vi "Main.vi"(11 "Module Admin":refnum<class "Delacor_lib_QMH_Cloneable Module Admin.lvclass">) -> ()   [LabVIEW 2020, in "Osciloscope.lvlib"]
doc: "This template is based off of the Queued Message Handler design pattern and the Queued Message Handler project template that ships with LabVIEW.\n\nThe main difference is that the queue is private to this module and communication between modules is performed via Broadcast and Request events.\n\nRequest events are wrapped in public API methods and are handled in the Event Handling Loop (EHL) of this VI. Any module can register for Broadcast events sent by this module. The EHL generates messages based on user interface actions.\n\nThe Message Handling Loop (MHL) processes messages generated by the EHL, or by other messages. The messages are string values, so new messages can be added easily to the Message Cases case structure in the MHL. Each message cluster can also provide an optional value for Message Data, which is a variant that can be converted to whatever message-specific data is required.\n_____\nBased on DQMH Project Template 6.0.0.91."
uses:
  Osciloscope.lvlib
  <vilib>/Delacor/Delacor QMH/Libraries/Cloneable Module Admin_class/Delacor_lib_QMH_Cloneable Module Admin.lvclass
  C:/Program Files (x86)/National Instruments/LabVIEW 2020/vi.lib/Delacor/Delacor QMH/Libraries/Module Admin_class/Delacor_lib_QMH_Module Admin.lvclass
  Module Data--cluster.ctl
  Classes/Osciloscope/Osciloscope.lvclass
  <vilib>/Delacor/Delacor QMH/Libraries/Message Queue_class/Delacor_lib_QMH_Message Queue.lvclass/Delacor_lib_QMH_Message Queue.ctl
  <vilib>/Delacor/Delacor QMH/Libraries/Cloneable Module Admin_class/Delacor_lib_QMH_Cloneable Module Admin.lvclass/Delacor_lib_QMH_Cloneable Module Admin.ctl
  Stop Argument--cluster.ctl
  <vilib>/Delacor/Delacor QMH/Libraries/Module Admin_class/Delacor_lib_QMH_Module Admin.lvclass/Delacor_lib_QMH_Module Admin.ctl
  Set Port Com Argument--cluster.ctl
  InicializarOsciloscopio Argument--cluster.ctl
  InitMethod Argument--cluster.ctl
  CloseMethod Argument--cluster.ctl
  MethodAutosetup Argument--cluster.ctl
  Method Configure Channel Argument--cluster.ctl
  Read Measurement Method Argument--cluster.ctl
  <vilib>/Utility/miscctls.llb/LVPointTypeDef.ctl
  Classes/Osciloscope/Osciloscope.lvclass/Osciloscope.ctl
  <vilib>/Delacor/Delacor QMH/Libraries/Message Queue_class/Delacor_lib_QMH_Enqueue Message (Single).vi
  <vilib>/Delacor/Delacor QMH/Libraries/Cloneable Module Admin_class/Delacor_lib_QMH_Get Module ID.vi
  <vilib>/Delacor/Delacor QMH/Libraries/Module Admin_class/Delacor_lib_QMH_Get External Launch.vi
  Classes/Osciloscope/Write COM.vi
  <vilib>/Utility/error.llb/Error Cluster From Error Code.vi
  <vilib>/ErrorRing/Error Ring.xnode
  <vilib>/Delacor/Delacor QMH/Libraries/Message Queue_class/Delacor_lib_QMH_Message Queue.lvclass
panel:
  out "error out":errorcluster
  out "Status":string
  in  "Simulate EHL Error":bool
  in  "Simulate MHL Error":bool
  # "Other QMH Modules communicate with this Module via its Public API (wrappers for its Request Events).\n\nThis Module communicates with other Modules via its Broadcast Events.\nAny module that wants to get these messages, just registers for this module's Broadcast events."
  # "This template is for the Delacor Modified Queued Message Handler design pattern.\n\nSee the block diagram for more information on how to use this template."
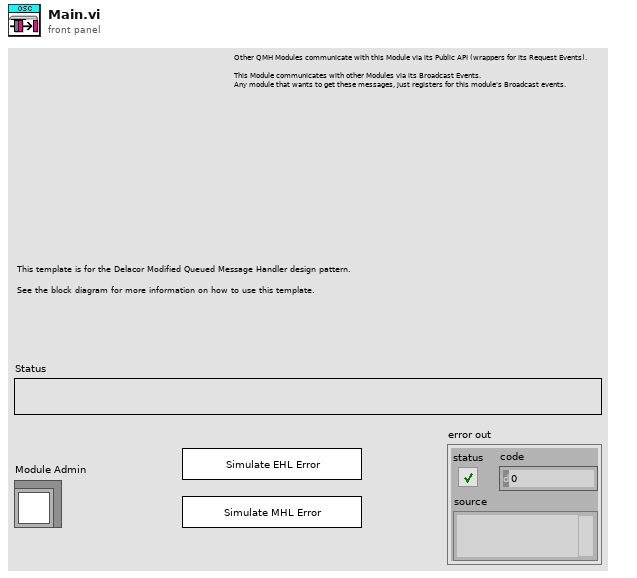
[diagram p1: front panel]
types:
  T1 = typedef "Osciloscope.lvlib/Request Events--cluster.ctl" = cluster{"Stop Module":refnum<user-event>, "Show Panel":refnum<user-event>, "Hide Panel":refnum<user-event>, "Show Diagram":refnum<user-event>, "Get Module Execution Status":refnum<user-event>, "Set Port Com":refnum<user-event>, "InicializarOsciloscopio":refnum<user-event>, "InitMethod":refnum<user-event>, "CloseMethod":refnum<user-event>, "MethodAutosetup":refnum<user-event>, "Method Configure Channel":refnum<user-event>, "Read Measurement Method":refnum<user-event>}
  T2 = typedef "Osciloscope.lvlib/Module Data--cluster.ctl" = cluster{"Status":string, "Com":refnum<visa-resource-name>, "Osciloscope.lvclass":refnum<class "Osciloscope.lvclass">}
  T3 = enum32{"invalid lock state", "Not Locked", "Locked (No Password)", "Password-protected"}
  T4 = typedef "Osciloscope.lvlib/Stop Argument--cluster.ctl" = cluster{"Module ID":i32, "Origin":string, "Exit via Stop Module Req?":bool, "Wait for Module to stop?":bool}
  T5 = typedef "Osciloscope.lvlib/Set Port Com Argument--cluster.ctl" = cluster{"Module ID":i32, "COM":refnum<visa-resource-name>}
  T6 = typedef "Osciloscope.lvlib/InicializarOsciloscopio Argument--cluster.ctl" = cluster{"Module ID":i32, "OsciloscopioName":string}
  T7 = typedef "Osciloscope.lvlib/InitMethod Argument--cluster.ctl" = cluster{"Module ID":i32, "Boolean":bool}
  T8 = typedef "Osciloscope.lvlib/CloseMethod Argument--cluster.ctl" = cluster{"Module ID":i32, "Boolean":bool}
  T9 = typedef "Osciloscope.lvlib/MethodAutosetup Argument--cluster.ctl" = cluster{"Module ID":i32, "Boolean":bool}
  T10 = typedef "Osciloscope.lvlib/Method Configure Channel Argument--cluster.ctl" = cluster{"Module ID":i32, "Boolean":bool}
  T11 = typedef "Osciloscope.lvlib/Read Measurement Method Argument--cluster.ctl" = cluster{"Module ID":i32, "Boolean":bool}
  T12 = typedef "LVPointTypeDef.ctl" = cluster{"Horizontal":i16, "Vertical":i16}
  T13 = enum32{"Invalid", "Standard", "Closed", "Hidden", "Minimized", "Maximized"}
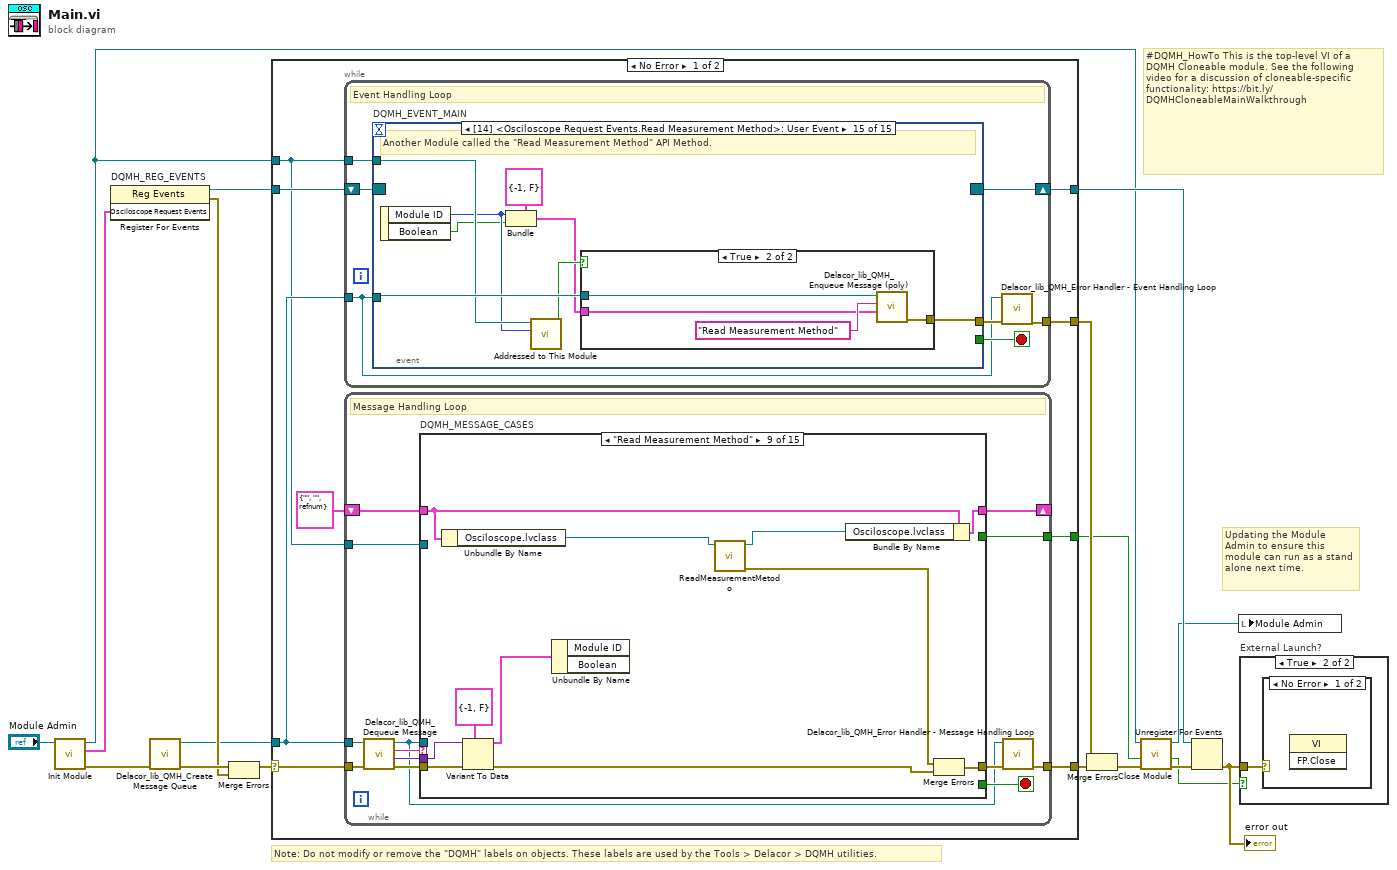
[diagram p0: block diagram]
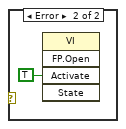
[diagram p3: hidden frame]
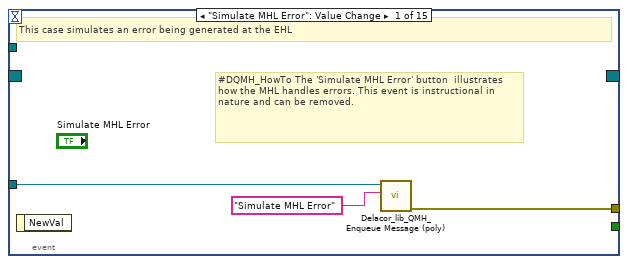
[diagram p4: hidden frame]
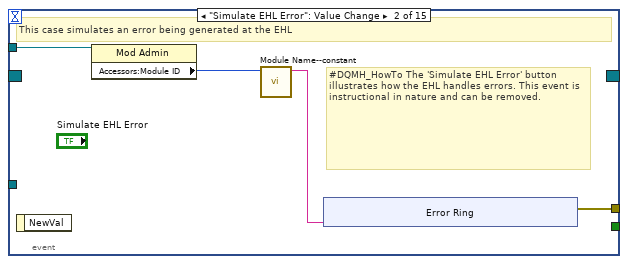
[diagram p5: hidden frame]
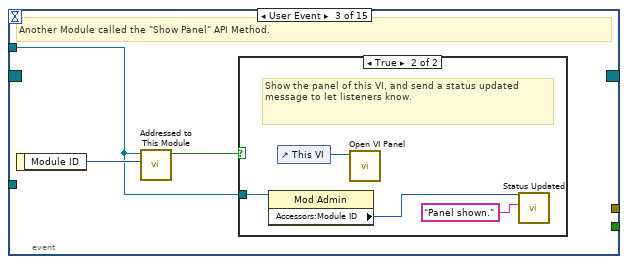
[diagram p6: hidden frame]
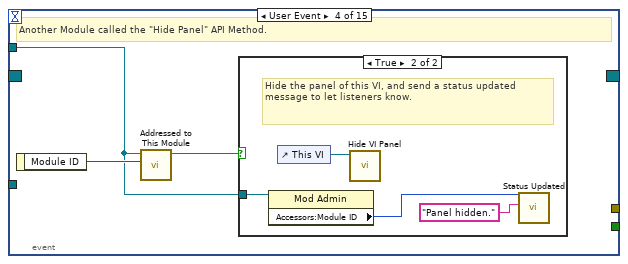
[diagram p8: hidden frame]
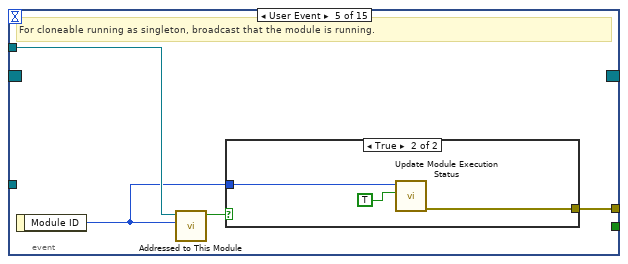
[diagram p10: hidden frame]
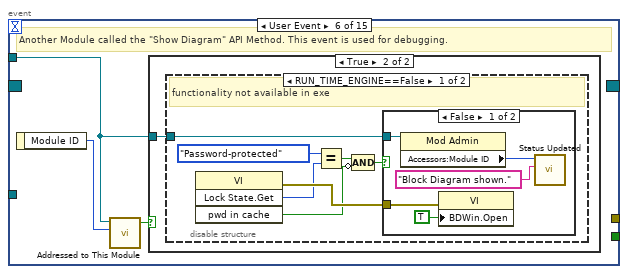
[diagram p12: hidden frame]
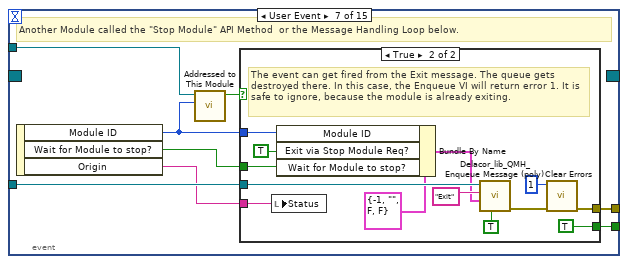
[diagram p16: hidden frame]
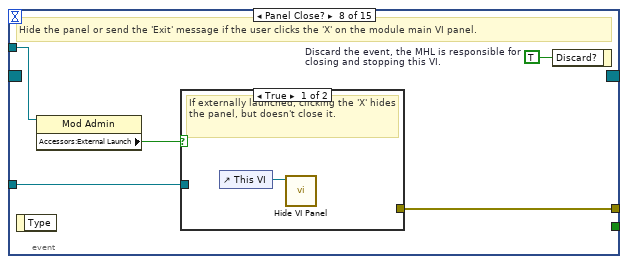
[diagram p18: hidden frame]
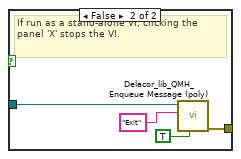
[diagram p19: hidden frame]
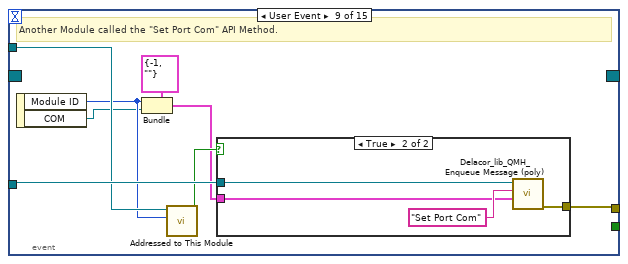
[diagram p20: hidden frame]
diagram:
  # "#DQMH_HowTo This is the top-level VI of a DQMH Cloneable module. See the following video for a discussion of cloneable-specific functionality: https://bit.ly/DQMHCloneableMainWalkthrough"
  # "Note: Do not modify or remove the \"DQMH\" labels on objects. These labels are used by the Tools > Delacor > DQMH utilities."
  # "Updating the Module Admin to ensure this module can run as a stand alone next time."
  n1 = call "Init Module.vi"("Cloneable Module Admin in"="Module Admin") -> ("error out"=w15:errorcluster, "Osciloscope Request Events"=w7:T1, "Cloneable Module Admin out"=w4:refnum<class "Delacor_lib_QMH_Cloneable Module Admin.lvclass">)  [unwired: 8 in]
  n2 = register-events "DQMH_REG_EVENTS"(w7) -> (reference out=w8:refnum<event-registration>, error out=w10:errorcluster)  [unwired: 2 in]
  n3 = call <vilib>:"Delacor_lib_QMH_Create Message Queue.vi"("error in"=w15) -> ("error out"=w12:errorcluster, "Message Queue"=w6:refnum<class "Delacor_lib_QMH_Message Queue.lvclass">)  [unwired: 9 in]
  n4 = Merge Errors(w12, w10) -> (w11:errorcluster)
  n5 = case shown="No Error" w11 {
    selector: w11 -> [w25 w384]
    tunnel: [w27 w383] -> w16
    tunnel: [w24 w391] -> w9
    tunnel: w8 -> [w22 w391]
    tunnel: w6 -> [w21 w382]
    tunnel: [w26 _] -> w17
    tunnel: w4 -> [w20 w387]
    tunnel: [w19 _] -> w2
    frame No Error {
      n6 = while {
        tunnel: w21 -> [w28]
        shift-right: [w31] -> w24
        shift-left: w22 -> [w32]
        tunnel: [w33] -> w26
        tunnel: w20 -> [w29]
        stop <- w30 stop-if-true
        # "Event Handling Loop"
        n7 = event "DQMH_EVENT_MAIN" shown="[14] <Osciloscope Request Events.Read Measurement Method>: User Event" {
          selector: w32 -> [_ _ _ _ _ _ _ _ _ _ _ _ _ _ _]
          dyn-events: [_ _ _ _ _ _ _ _ _ _ _ _ _ _ _] -> w31
          timeout: _ -> [_ _ _ _ _ _ _ _ _ _ _ _ _ _ _]
          tunnel: [_ _ _ _ _ _ w89 _ _ _ _ _ _ _ _] -> w30
          tunnel: w28 -> [w36 _ _ _ _ _ w92 w108 w124 w136 w148 w160 w172 w184 w196]
          tunnel: [w37 w41 _ _ w66 _ w93 w111 w117 w129 w141 w153 w165 w177 w189] -> w34
          tunnel: w29 -> [_ w40 w49 w56 w64 w70 w91 w109 w122 w134 w146 w158 w170 w182 w194]
          event "Simulate MHL Error": Value Change {
            # "#DQMH_HowTo The 'Simulate MHL Error' button  illustrates how the MHL handles errors. This event is instructional in nature and can be removed."
            # "This case simulates an error being generated at the EHL"
            n8 = event-data() -> ()  [unwired: 1 in, 1 out]
            n9 = call-poly <vilib>:"Delacor_lib_QMH_Enqueue Message (poly).vi"("Message"="Simulate MHL Error", "Message Queue in"=w36) -> ("error out"=w37:errorcluster)  [unwired: 8 in, 1 out]
          }
          event "Simulate EHL Error": Value Change {
            # "#DQMH_HowTo The 'Simulate EHL Error' button  illustrates how the EHL handles errors. This event is instructional in nature and can be removed."
            # "This case simulates an error being generated at the EHL"
            n10 = event-data() -> ()  [unwired: 1 in, 1 out]
            n11 = property class="Mod Admin"(reference=w40) -> ("Accessors:Module ID"=w39:i32)  [unwired: 1 in, 2 out]
            n12 = call "Module Name--constant.vi"("Module ID"=w39) -> ("Module Name"=w38:string)  [unwired: 10 in]
            n13 = xnode "Error Ring"("parameter 0"=w38) -> ("error out"=w41:errorcluster)
          }
          event User Event {
            # "Another Module called the \"Show Panel\" API Method."
            n14 = event-data() -> ("Module ID"=w50:i32)  [unwired: 1 in]
            n15 = call "Addressed to This Module.vi"("Module ID from Argument"=w50, "Module Admin"=w49) -> ("Addressed to this instance?"=w51:bool)  [unwired: 8 in, 1 out]
            n16 = case shown="True" w51 {
              tunnel: w49 -> [_ w53]
              frame False {
              }
              frame True {
                # "Show the panel of this VI, and send a status updated message to let listeners know."
                n17 = property class="Mod Admin"(reference=w53) -> ("Accessors:Module ID"=w52:i32)  [unwired: 1 in, 2 out]
                n18 = control-ref of="This VI"() -> (w55:refnum<vi>)
                n19 = call "Open VI Panel.vi"("VI"=w55) -> ()  [unwired: 10 in, 1 out]
                n20 = call "Status Updated.vi"("Status"="Panel shown." ("format string"), "Module ID"=w52) -> ()  [unwired: 9 in, 1 out]
              }
            }
          }
          event User Event {
            # "Another Module called the \"Hide Panel\" API Method."
            n21 = event-data() -> ("Module ID"=w57:i32)  [unwired: 1 in]
            n22 = call "Addressed to This Module.vi"("Module ID from Argument"=w57, "Module Admin"=w56) -> ("Addressed to this instance?"=w58:bool)  [unwired: 8 in, 1 out]
            n23 = case shown="True" w58 {
              tunnel: w56 -> [_ w60]
              frame False {
              }
              frame True {
                # "Hide the panel of this VI, and send a status updated message to let listeners know."
                n24 = property class="Mod Admin"(reference=w60) -> ("Accessors:Module ID"=w59:i32)  [unwired: 1 in, 2 out]
                n25 = control-ref of="This VI"() -> (w62:refnum<vi>)
                n26 = call "Hide VI Panel.vi"("VI"=w62) -> ()  [unwired: 10 in, 1 out]
                n27 = call "Status Updated.vi"("Status"="Panel hidden." ("format string"), "Module ID"=w59) -> ()  [unwired: 9 in, 1 out]
              }
            }
          }
          event User Event {
            # "For cloneable running as singleton, broadcast that the module is running."
            n28 = event-data() -> ("Module ID"=w63:i32)  [unwired: 1 in]
            n29 = call "Addressed to This Module.vi"("Module ID from Argument"=w63, "Module Admin"=w64) -> ("Addressed to this instance?"=w65:bool)  [unwired: 8 in, 1 out]
            n30 = case shown="True" w65 {
              tunnel: [_ w69] -> w66
              tunnel: w63 -> [_ w68]
              frame False {
              }
              frame True {
                n31 = call "Update Module Execution Status.vi"("Running?"=TRUE, "Module ID"=w68) -> ("error out"=w69:errorcluster)  [unwired: 9 in]
              }
            }
          }
          event User Event {
            # "Another Module called the \"Show Diagram\" API Method. This event is used for debugging."
            n32 = event-data() -> ("Module ID"=w71:i32)  [unwired: 1 in]
            n33 = call "Addressed to This Module.vi"("Module ID from Argument"=w71, "Module Admin"=w70) -> ("Addressed to this instance?"=w72:bool)  [unwired: 8 in, 1 out]
            n34 = case shown="True" w72 {
              tunnel: w70 -> [_ w73]
              frame False {
              }
              frame True {
                n35 = disable-structure shown="RUN_TIME_ENGINE==False" {
                  disable-tunnel: w73 -> [w74 _]
                  frame condition #0 (active) {
                    # "functionality not available in exe"
                    n36 = invoke class="VI" method="Lock State.Get"() -> (error out=w80:errorcluster, "Get Lock State"=w79:T3, "pwd in cache"=w76:bool)  [unwired: 4 in, 1 out]
                    n37 = Equal?(x=T3."Password-protected", y=w79) -> (x = y?=w77:bool)
                    n38 = Compound Arithmetic op=AND(w77, invert w76) -> (w75:bool)
                    n39 = case shown="False" w75 {
                      tunnel: w80 -> [w85 _]
                      tunnel: w74 -> [w82 _]
                      frame False {
                        n40 = property class="Mod Admin"(reference=w82) -> ("Accessors:Module ID"=w81:i32)  [unwired: 1 in, 2 out]
                        n41 = property class="VI"(error in=w85, "BDWin.Open"=TRUE ("Block Diagram Window:Open")) -> ()  [unwired: 1 in, 2 out]
                        n42 = call "Status Updated.vi"("Status"="Block Diagram shown." ("format string"), "Module ID"=w81) -> ()  [unwired: 9 in, 1 out]
                      }
                      frame True {
                        # "Password-protected VI, and the password is not in the cache. Do not show the diagram."
                      }
                    }
                  }
                  frame condition #1 {
                  }
                }
              }
            }
          }
          event User Event {
            # "Another Module called the \"Stop Module\" API Method  or the Message Handling Loop below."
            n43 = event-data() -> ("Module ID"=w87:i32, "Wait for Module to stop?"=w88:bool, "Origin"=w86:string)  [unwired: 1 in]
            n44 = call "Addressed to This Module.vi"("Module ID from Argument"=w87, "Module Admin"=w91) -> ("Addressed to this instance?"=w90:bool)  [unwired: 8 in, 1 out]
            n45 = case shown="True" w90 {
              tunnel: [_ w105] -> w93
              tunnel: w92 -> [_ w101]
              tunnel: [_ TRUE] -> w89
              tunnel: w88 -> [_ w96]
              tunnel: w87 -> [_ w98]
              tunnel: w86 -> [_ w94]
              frame False {
              }
              frame True {
                # "The event can get fired from the Exit message. The queue gets destroyed there. In this case, the Enqueue VI will return error 1. It is safe to ignore, because the module is already exiting."
                n46 = local write "Status"(w94) -> ()
                n47 = Bundle By Name(cluster=T4 {"Module ID"=-1, "Origin"="", "Exit via Stop Module Req?"=FALSE, "Wait for Module to stop?"=FALSE} ("Stop Argument"), "Module ID"=w98, "Exit via Stop Module Req?"=TRUE, "Wait for Module to stop?"=w96) -> (w95:T4)
                n48 = call-poly <vilib>:"Delacor_lib_QMH_Enqueue Message (poly).vi"("Priority Message? (F)"=TRUE, "Message Data"=w95, "Message"="Exit", "Message Queue in"=w101) -> ("error out"=w106:errorcluster)  [unwired: 6 in, 1 out]
                n49 = call <vilib>:"Clear Errors.vi"("error in (no error)"=w106, "specific error code to clear (0: all)"=1) -> ("error out"=w105:errorcluster)  [unwired: 4 in, 1 out]
              }
            }
          }
          event Panel Close? {
            w110 = TRUE  # Discard the event, the MHL is responsible for closing and stopping this VI.
            # "Hide the panel or send the 'Exit' message if the user clicks the 'X' on the module main VI panel."
            n50 = event-data() -> ()  [unwired: 1 in, 1 out]
            n51 = property class="Mod Admin"(reference=w109) -> ("Accessors:External Launch"=w107:bool)  [unwired: 1 in, 2 out]
            n52 = case shown="True" w107 {
              tunnel: w108 -> [_ w115]
              tunnel: [_ w116] -> w111
              frame True {
                # "If externally launched, clicking the 'X' hides the panel, but doesn't close it."
                n53 = control-ref of="This VI"() -> (w112:refnum<vi>)
                n54 = call "Hide VI Panel.vi"("VI"=w112) -> ()  [unwired: 10 in, 1 out]
              }
              frame False {
                # "If run as a stand-alone VI, clicking the panel 'X' stops the VI."
                n55 = call-poly <vilib>:"Delacor_lib_QMH_Enqueue Message (poly).vi"("Priority Message? (F)"=TRUE, "Message"="Exit", "Message Queue in"=w115) -> ("error out"=w116:errorcluster)  [unwired: 7 in, 1 out]
              }
            }
            n56 = event-data("Discard?"=w110) -> ()  [unwired: 1 in, 1 out]
          }
          event User Event {
            # "Another Module called the \"Set Port Com\" API Method."
            n57 = event-data() -> ("Module ID"=w119:i32, "COM"=w118:refnum<visa-resource-name>)  [unwired: 1 in]
            n58 = Bundle(cluster=T5 {"Module ID"=-1, "COM"=""} ("Set Port Com Argument"), "Module ID"=w119, "COM"=w118) -> (w120:T5)
            n59 = call "Addressed to This Module.vi"("Module ID from Argument"=w119, "Module Admin"=w122) -> ("Addressed to this instance?"=w123:bool)  [unwired: 8 in, 1 out]
            n60 = case shown="True" w123 {
              tunnel: w124 -> [_ w128]
              tunnel: w120 -> [_ w126]
              tunnel: [_ w125] -> w117
              frame False {
              }
              frame True {
                n61 = call-poly <vilib>:"Delacor_lib_QMH_Enqueue Message (poly).vi"("Message Data"=w126, "Message"="Set Port Com", "Message Queue in"=w128) -> ("error out"=w125:errorcluster)  [unwired: 7 in, 1 out]
              }
            }
          }
          event User Event {
            # "Another Module called the \"InicializarOsciloscopio\" API Method."
            n62 = event-data() -> ("Module ID"=w131:i32, "OsciloscopioName"=w130:string)  [unwired: 1 in]
            n63 = Bundle(cluster=T6 {"Module ID"=-1, "OsciloscopioName"=""} ("InicializarOsciloscopio Argument"), "Module ID"=w131, "OsciloscopioName"=w130) -> (w132:T6)
            n64 = call "Addressed to This Module.vi"("Module ID from Argument"=w131, "Module Admin"=w134) -> ("Addressed to this instance?"=w135:bool)  [unwired: 8 in, 1 out]
            n65 = case shown="True" w135 {
              tunnel: w136 -> [_ w140]
              tunnel: w132 -> [_ w138]
              tunnel: [_ w137] -> w129
              frame False {
              }
              frame True {
                n66 = call-poly <vilib>:"Delacor_lib_QMH_Enqueue Message (poly).vi"("Message Data"=w138, "Message"="InicializarOsciloscopio", "Message Queue in"=w140) -> ("error out"=w137:errorcluster)  [unwired: 7 in, 1 out]
              }
            }
          }
          event User Event {
            # "Another Module called the \"InitMethod\" API Method."
            n67 = event-data() -> ("Module ID"=w143:i32, "Boolean"=w142:bool)  [unwired: 1 in]
            n68 = Bundle(cluster=T7 {"Module ID"=-1, "Boolean"=FALSE} ("InitMethod Argument"), "Module ID"=w143, "Boolean"=w142) -> (w144:T7)
            n69 = call "Addressed to This Module.vi"("Module ID from Argument"=w143, "Module Admin"=w146) -> ("Addressed to this instance?"=w147:bool)  [unwired: 8 in, 1 out]
            n70 = case shown="True" w147 {
              tunnel: w148 -> [_ w152]
              tunnel: w144 -> [_ w150]
              tunnel: [_ w149] -> w141
              frame False {
              }
              frame True {
                n71 = call-poly <vilib>:"Delacor_lib_QMH_Enqueue Message (poly).vi"("Message Data"=w150, "Message"="InitMethod", "Message Queue in"=w152) -> ("error out"=w149:errorcluster)  [unwired: 7 in, 1 out]
              }
            }
          }
          event User Event {
            # "Another Module called the \"CloseMethod\" API Method."
            n72 = event-data() -> ("Module ID"=w155:i32, "Boolean"=w154:bool)  [unwired: 1 in]
            n73 = Bundle(cluster=T8 {"Module ID"=-1, "Boolean"=FALSE} ("CloseMethod Argument"), "Module ID"=w155, "Boolean"=w154) -> (w156:T8)
            n74 = call "Addressed to This Module.vi"("Module ID from Argument"=w155, "Module Admin"=w158) -> ("Addressed to this instance?"=w159:bool)  [unwired: 8 in, 1 out]
            n75 = case shown="True" w159 {
              tunnel: w160 -> [_ w164]
              tunnel: w156 -> [_ w162]
              tunnel: [_ w161] -> w153
              frame False {
              }
              frame True {
                n76 = call-poly <vilib>:"Delacor_lib_QMH_Enqueue Message (poly).vi"("Message Data"=w162, "Message"="CloseMethod", "Message Queue in"=w164) -> ("error out"=w161:errorcluster)  [unwired: 7 in, 1 out]
              }
            }
          }
          event User Event {
            # "Another Module called the \"MethodAutosetup\" API Method."
            n77 = event-data() -> ("Module ID"=w167:i32, "Boolean"=w166:bool)  [unwired: 1 in]
            n78 = Bundle(cluster=T9 {"Module ID"=-1, "Boolean"=FALSE} ("MethodAutosetup Argument"), "Module ID"=w167, "Boolean"=w166) -> (w168:T9)
            n79 = call "Addressed to This Module.vi"("Module ID from Argument"=w167, "Module Admin"=w170) -> ("Addressed to this instance?"=w171:bool)  [unwired: 8 in, 1 out]
            n80 = case shown="True" w171 {
              tunnel: w172 -> [_ w176]
              tunnel: w168 -> [_ w174]
              tunnel: [_ w173] -> w165
              frame False {
              }
              frame True {
                n81 = call-poly <vilib>:"Delacor_lib_QMH_Enqueue Message (poly).vi"("Message Data"=w174, "Message"="MethodAutosetup", "Message Queue in"=w176) -> ("error out"=w173:errorcluster)  [unwired: 7 in, 1 out]
              }
            }
          }
          event User Event {
            # "Another Module called the \"Method Configure Channel\" API Method."
            n82 = event-data() -> ("Module ID"=w179:i32, "Boolean"=w178:bool)  [unwired: 1 in]
            n83 = Bundle(cluster=T10 {"Module ID"=-1, "Boolean"=FALSE} ("Method Configure Channel Argument"), "Module ID"=w179, "Boolean"=w178) -> (w180:T10)
            n84 = call "Addressed to This Module.vi"("Module ID from Argument"=w179, "Module Admin"=w182) -> ("Addressed to this instance?"=w183:bool)  [unwired: 8 in, 1 out]
            n85 = case shown="True" w183 {
              tunnel: w184 -> [_ w188]
              tunnel: w180 -> [_ w186]
              tunnel: [_ w185] -> w177
              frame False {
              }
              frame True {
                n86 = call-poly <vilib>:"Delacor_lib_QMH_Enqueue Message (poly).vi"("Message Data"=w186, "Message"="Method Configure Channel", "Message Queue in"=w188) -> ("error out"=w185:errorcluster)  [unwired: 7 in, 1 out]
              }
            }
          }
          event User Event {
            # "Another Module called the \"Read Measurement Method\" API Method."
            n87 = event-data() -> ("Module ID"=w191:i32, "Boolean"=w190:bool)  [unwired: 1 in]
            n88 = Bundle(cluster=T11 {"Module ID"=-1, "Boolean"=FALSE} ("Read Measurement Method Argument"), "Module ID"=w191, "Boolean"=w190) -> (w192:T11)
            n89 = call "Addressed to This Module.vi"("Module ID from Argument"=w191, "Module Admin"=w194) -> ("Addressed to this instance?"=w195:bool)  [unwired: 8 in, 1 out]
            n90 = case shown="True" w195 {
              tunnel: w196 -> [_ w200]
              tunnel: w192 -> [_ w198]
              tunnel: [_ w197] -> w189
              frame False {
              }
              frame True {
                n91 = call-poly <vilib>:"Delacor_lib_QMH_Enqueue Message (poly).vi"("Message Data"=w198, "Message"="Read Measurement Method", "Message Queue in"=w200) -> ("error out"=w197:errorcluster)  [unwired: 7 in, 1 out]
              }
            }
          }
        }
        n92 = call-dynamic "Delacor_lib_QMH_Error Handler - Event Handling Loop.vi"("error in"=w34, "Message Queue in"=w28) -> ("dup error in"=w33:errorcluster)  [unwired: 8 in, 1 out]
      }
      n93 = while {
        tunnel: w21 -> [w204]
        shift-right: [w208] -> _
        shift-left: T2 {"Status"="", "Com"="", "Osciloscope.lvclass"=refnum} ("Data Cluster") -> [w209]
        tunnel: w25 -> [w212]
        tunnel: [w210] -> w27
        tunnel: w20 -> [w202]
        tunnel: [w201] -> w19
        stop <- w207 stop-if-true
        # "Message Handling Loop"
        n94 = call-dynamic "Delacor_lib_QMH_Dequeue Message.vi"("error in"=w212, "Message Queue in"=w204) -> ("error out"=w211:errorcluster, "Message Data"=w205:variant, "Message"=w206:string, "Message Queue out"=w203:refnum<class "Delacor_lib_QMH_Message Queue.lvclass">)  [unwired: 6 in]
        n95 = case "DQMH_MESSAGE_CASES" shown="\"Read Measurement Method\"" w206 {
          selector: w206 -> [_ _ _ _ _ _ _ _ _ _ _ _ _ _ w369]
          tunnel: w203 -> [_ _ _ _ _ _ _ _ _ _ _ w320 _ w359 _]
          tunnel: w211 -> [w233 w237 w245 w260 w269 w280 w291 w302 w313 w316 w318 w329 w342 w365 w371]
          tunnel: [w231 w237 w244 w251 w268 w272 w287 w296 w305 w315 w318 w325 w341 w362 w372] -> w213
          tunnel: w209 -> [w224 w236 w240 w259 w263 w276 w284 w297 w308 w314 w317 w324 w339 w358 w370]
          tunnel: [w223 w236 w238 w254 w262 w275 w285 w298 w309 w314 w317 w324 w339 w358 w370] -> w208
          tunnel: [_ _ _ _ _ _ _ _ _ _ _ _ _ w357 _] -> w207
          tunnel: w205 -> [_ _ w243 w258 w267 w279 w290 w301 w312 _ _ w323 _ w355 _]
          tunnel: w202 -> [w219 _ _ _ _ _ _ _ _ _ _ w322 w337 w351 w367]
          tunnel: [_ _ _ _ _ _ _ _ _ _ _ _ _ w353 _] -> w201
          frame "Initialize" {
            w216 = "Initial Message" ("Initial Message")
            # "Initialize - Any operation that needs to be done before the module can receive messages. Synchronize Caller Events.vi will inform Start Module.vi that the module has launched and is ready to receive messages. Module Did Init.vi will broadcast that the module initialized."
            n96 = call "Synchronize Caller Events.vi"("error in (no error)"=w233, "Module Admin"=w219) -> ("error out"=w232:errorcluster, "Module Admin out"=w218:refnum<class "Delacor_lib_QMH_Cloneable Module Admin.lvclass">)  [unwired: 8 in]
            n97 = call "GetClass.vi"() -> ("Classes"=w214:string[])  [unwired: 11 in]
            n98 = property class="Mod Admin"(reference=w218) -> ("Accessors:Module ID"=w215:i32, "Accessors:External Launch"=w220:bool)  [unwired: 1 in, 2 out]
            n99 = call "OsciloscopesTypes.vi"("Osciloscopes"=w214, "Module ID"=w215) -> ()  [unwired: 9 in, 1 out]
            n100 = call "Module Name--constant.vi"("Module ID"=w215) -> ("Module Name"=w228:string)  [unwired: 10 in]
            n101 = property class="VI"("Front Panel.Title"=w228) -> (reference out=w230:refnum<vi>, error out=w235:errorcluster)  [unwired: 2 in]
            n102 = Select(t=T13."Hidden" ("State"), s=w220, f=T13."Standard" ("State")) -> (s? t:f=w225:T13)
            n103 = invoke class="VI" method="FP.Open"(reference=w230, error in=w235, "State"=w225) -> (reference out=w229:refnum<vi>, error out=w234:errorcluster)  [unwired: 2 in, 3 out]
            n104 = call "Module Name--constant.vi"("Module ID"=w215) -> ("Module Name"=w221:string)  [unwired: 10 in]
            n105 = Bundle By Name(cluster=w224, "Status"=w216) -> (w223:T2)
            n106 = invoke class="VI" method="FP.Center"(reference=w229, error in=w234) -> ()  [unwired: 1 in, 3 out]
            n107 = property on="Pane" class="Pane"("Origin"=T12 {"Horizontal"=0, "Vertical"=0}) -> ()  [unwired: 2 in, 2 out]
            n108 = call "Module Did Init.vi"("error in (no error)"=w232, "Initialized?"=TRUE, "Origin"=w221, "Module ID"=w215) -> ("error out"=w231:errorcluster)  [unwired: 7 in]
            "Status" <- w216
          }
          frame "---Module Specific---" {
            # "Separator -- The following cases handle messages specific to this Module."
          }
          frame "Set Port Com" {
            n109 = Variant To Data(error in=w245, type=T5 {"Module ID"=-1, "COM"=""} ("Set Port Com Argument"), Variant=w243) -> (data=w241:T5, error out=w244:errorcluster)
            n110 = Unbundle By Name(w241) -> ("COM"=w239:refnum<visa-resource-name>)
            n111 = in-place {
              in-place-border: w239 -> [w247]
              n112 = in-place-cluster #1(w240) -> ("Osciloscope.lvclass"=w248:refnum<class "Osciloscope.lvclass">)
              n113 = property class="Osciloscope.lvclass"(reference=w248, "Accessors:COM"=w247) -> (reference out=w246:refnum<class "Osciloscope.lvclass">)  [unwired: 1 in, 1 out]
              n114 = in-place-cluster #1("Osciloscope.lvclass"=w246) -> (w238:T2)
            }
          }
          frame "InicializarOsciloscopio" {
            n115 = Variant To Data(error in=w260, type=T6 {"Module ID"=-1, "OsciloscopioName"=""} ("InicializarOsciloscopio Argument"), Variant=w258) -> (data=w256:T6, error out=w249:errorcluster)
            n116 = Unbundle By Name(w256) -> ("OsciloscopioName"=w255:string)
            n117 = call "SetClassInstance.vi"("TypeOsciloscope"=w255) -> ("OsciloscopeName"=w253:refnum<class "Osciloscope.lvclass">)  [unwired: 10 in]
            n118 = call "Pattern.vi"("Osciloscope in"=w253) -> ("error out"=w250:errorcluster, "Osciloscope out"=w252:refnum<class "Osciloscope.lvclass">)  [unwired: 9 in]
            n119 = Bundle By Name(cluster=w259, "Osciloscope.lvclass"=w252) -> (w254:T2)
            n120 = Merge Errors(w250, w249) -> (w251:errorcluster)
          }
          frame "InitMethod" {
            n121 = Variant To Data(error in=w269, type=T7 {"Module ID"=-1, "Boolean"=FALSE} ("InitMethod Argument"), Variant=w267) -> (data=w265:T7, error out=w268:errorcluster)
            n122 = Unbundle By Name(w263) -> ("Osciloscope.lvclass"=w264:refnum<class "Osciloscope.lvclass">)
            n123 = Unbundle By Name(w265) -> ()  [unwired: 2 out]
            n124 = call-dynamic "MetodoInit.vi"("Osciloscope in"=w264) -> ("Osciloscope out"=w261:refnum<class "Osciloscope.lvclass">)  [unwired: 8 in, 2 out]
            n125 = Bundle By Name(cluster=w263, "Osciloscope.lvclass"=w261) -> (w262:T2)
          }
          frame "CloseMethod" {
            n126 = Variant To Data(error in=w280, type=T8 {"Module ID"=-1, "Boolean"=FALSE} ("CloseMethod Argument"), Variant=w279) -> (data=w277:T8, error out=w270:errorcluster)
            n127 = Unbundle By Name(w276) -> ("Osciloscope.lvclass"=w274:refnum<class "Osciloscope.lvclass">)
            n128 = Unbundle By Name(w277) -> ()  [unwired: 2 out]
            n129 = call-dynamic "CloseMetodo.vi"("Osciloscope in"=w274) -> ("error out"=w271:errorcluster, "Osciloscope out"=w273:refnum<class "Osciloscope.lvclass">)  [unwired: 9 in]
            n130 = Bundle By Name(cluster=w276, "Osciloscope.lvclass"=w273) -> (w275:T2)
            n131 = Merge Errors(w271, w270) -> (w272:errorcluster)
          }
          frame "MethodAutosetup" {
            n132 = Unbundle By Name(w284) -> ("Osciloscope.lvclass"=w283:refnum<class "Osciloscope.lvclass">)
            n133 = Variant To Data(error in=w291, type=T9 {"Module ID"=-1, "Boolean"=FALSE} ("MethodAutosetup Argument"), Variant=w290) -> (data=w288:T9, error out=w286:errorcluster)
            n134 = Unbundle By Name(w288) -> ()  [unwired: 2 out]
            n135 = call-dynamic "AutoSetUpMetodo.vi"("Osciloscope in"=w283) -> ("error out"=w281:errorcluster, "Osciloscope out"=w282:refnum<class "Osciloscope.lvclass">)  [unwired: 8 in, 1 out]
            n136 = Bundle By Name(cluster=w284, "Osciloscope.lvclass"=w282) -> (w285:T2)
            n137 = Merge Errors(w281, w286) -> (w287:errorcluster)
          }
          frame "Method Configure Channel" {
            n138 = Unbundle By Name(w297) -> ("Osciloscope.lvclass"=w294:refnum<class "Osciloscope.lvclass">)
            n139 = Variant To Data(error in=w302, type=T10 {"Module ID"=-1, "Boolean"=FALSE} ("Method Configure Channel Argument"), Variant=w301) -> (data=w299:T10, error out=w295:errorcluster)
            n140 = Unbundle By Name(w299) -> ()  [unwired: 2 out]
            n141 = call-dynamic "ConfChannelMetodo.vi"("Osciloscope in"=w294) -> ("error out"=w292:errorcluster, "Osciloscope out"=w293:refnum<class "Osciloscope.lvclass">)  [unwired: 8 in, 1 out]
            n142 = Bundle By Name(cluster=w297, "Osciloscope.lvclass"=w293) -> (w298:T2)
            n143 = Merge Errors(w292, w295) -> (w296:errorcluster)
          }
          frame "Read Measurement Method" {
            n144 = Unbundle By Name(w308) -> ("Osciloscope.lvclass"=w307:refnum<class "Osciloscope.lvclass">)
            n145 = Variant To Data(error in=w313, type=T11 {"Module ID"=-1, "Boolean"=FALSE} ("Read Measurement Method Argument"), Variant=w312) -> (data=w310:T11, error out=w304:errorcluster)
            n146 = Unbundle By Name(w310) -> ()  [unwired: 2 out]
            n147 = call-dynamic "ReadMeasurementMetodo.vi"("Osciloscope in"=w307) -> ("error out"=w303:errorcluster, "Osciloscope out"=w306:refnum<class "Osciloscope.lvclass">)  [unwired: 8 in, 1 out]
            n148 = Bundle By Name(cluster=w308, "Osciloscope.lvclass"=w306) -> (w309:T2)
            n149 = Merge Errors(w303, w304) -> (w305:errorcluster)
          }
          frame "---Copy This Frame---" {
            # "Duplicate this frame when creating new messages.  Change this comment in the duplicated frame to describe this message."
            n150 = Merge Errors(w316) -> (w315:errorcluster)
          }
          frame "---Exit and Error Handling---" {
            # "Separator - the following cases handle errors and exit messages."
          }
          frame "Error" {
            # "#CodeRecommended - If you ever change the name of this \"Error\" message, you'll need to update the name in the Check Loop Error.vi as well."
            # "#CodeRecommended - If the module is running in standalone mode (External Launch = FALSE), this code will pop up an error dialog and call the 'Exit' message if an error occurs. Add more fine-grained error handling here."
            # "Error - Check the error message data and respond accordingly. This message is sent by the \"Error Handler\" VIs at the end of each loop in this application."
            n151 = property class="Mod Admin"(reference=w322) -> ("Accessors:External Launch"=w321:bool, "Accessors:Module ID"=w319:i32)  [unwired: 1 in, 2 out]
            n152 = Variant To Data(error in=w329, type=errorcluster {"status"=FALSE, "code"=0, "source"=""} ("error constant"), Variant=w323) -> (data=w330:errorcluster, error out=w327:errorcluster)
            n153 = call "Error Reported.vi"("Error"=w330, "Module ID"=w319) -> ()  [unwired: 9 in, 1 out]
            n154 = case shown="False" w321 {
              tunnel: [w335 _] -> w326
              tunnel: w320 -> [w333 _]
              tunnel: w330 -> [w334 _]
              frame False {
                # "If the module is running standalone, then pop up an error dialog and call the \"Exit\" message."
                n155 = call <vilib>:"Simple Error Handler.vi"("error in (no error)"=w334) -> ()  [unwired: 4 in, 5 out]
                n156 = call-poly <vilib>:"Delacor_lib_QMH_Enqueue Message (poly).vi"("Priority Message? (F)"=TRUE, "Message"="Exit", "Message Queue in"=w333) -> ("error out"=w335:errorcluster)  [unwired: 7 in, 1 out]
              }
              frame True {
                # "If the module was launched externally, calling the Error Reported broadcast VI is the only action performed by the \"Error\" message. The module's caller can then process the error appropriately."
              }
            }
            n157 = Merge Errors(w327, w326) -> (w325:errorcluster)
            n158 = local write "error out"(w325) -> ()
          }
          frame "Simulate MHL Error" {
            # "#DQMH_HowTo The 'Simulate MHL Error' button  illustrates how the MHL handles errors. This event is instructional in nature and can be removed."
            # "Simulate an error occurring at the MHL"
            n159 = property class="Mod Admin"(reference=w337) -> ("Accessors:Module ID"=w338:i32)  [unwired: 1 in, 2 out]
            n160 = call "Module Name--constant.vi"("Module ID"=w338) -> ("Module Name"=w336:string)  [unwired: 10 in]
            n161 = xnode "Error Ring"("parameter 0"=w336) -> ("error out"=w340:errorcluster)
            n162 = Merge Errors(w342, w340) -> (w341:errorcluster)
          }
          frame "Exit" {
            w356 = 91  # 91: not all Exit messages will have an argument
            w357 = TRUE  # Stop the VI
            # "Release the message queue reference"
            # "#CodeNeeded - Add any required cleanup code here."
            # "Exit - Exit the application."
            n163 = Variant To Data(error in=w365, type=T4 {"Module ID"=-1, "Origin"="", "Exit via Stop Module Req?"=FALSE, "Wait for Module to stop?"=FALSE} ("Stop Argument"), Variant=w355) -> (data=w352:T4, error out=w360:errorcluster)
            n164 = call <vilib>:"Clear Errors.vi"("error in (no error)"=w360, "specific error code to clear (0: all)"=w356) -> ("error out"=w364:errorcluster)  [unwired: 4 in, 1 out]
            n165 = control-ref of="This VI"() -> (w350:refnum<vi>)
            n166 = call-dynamic "Delacor_lib_QMH_Release Message Queue.vi"("error in"=w364, "Message Queue"=w359) -> ("error out"=w363:errorcluster)  [unwired: 9 in]
            n167 = call "Handle Exit.vi"("Stop Argument"=w352, "Module Admin in"=w351, "VI reference"=w350) -> ("error out"=w361:errorcluster, "Wait for Stop?"=w353:bool)  [unwired: 7 in]
            n168 = Merge Errors(w363, w361) -> (w362:errorcluster)
          }
          frame Default {
            # "'Default' case only runs if there is a message that isn't defined in any of the other cases.  Output a programming error."
            n169 = property class="Mod Admin"(reference=w367) -> ("Accessors:Module ID"=w366:i32)  [unwired: 1 in, 2 out]
            n170 = call "Module Name--constant.vi"("Module ID"=w366) -> ("Module Name"=w368:string)  [unwired: 10 in]
            n171 = xnode "Error Ring"("parameter 0"=w369, "parameter 1"=w368) -> ("error out"=w373:errorcluster)
            n172 = Merge Errors(w371, w373) -> (w372:errorcluster)
          }
        }
        n173 = call-dynamic "Delacor_lib_QMH_Error Handler - Message Handling Loop.vi"("error in"=w213, "Message Queue in"=w203) -> ("dup error in"=w210:errorcluster)  [unwired: 8 in, 1 out]
      }
    }
    frame Error {
      n174 = call "Synchronize Caller Events.vi"("Module Admin"=w387) -> ("Module Admin out"=w386:refnum<class "Delacor_lib_QMH_Cloneable Module Admin.lvclass">)  [unwired: 9 in, 1 out]
      n175 = property class="Mod Admin"(reference=w386) -> ("Accessors:Module ID"=w385:i32)  [unwired: 1 in, 2 out]
      n176 = call-dynamic "Delacor_lib_QMH_Release Message Queue.vi"("error in"=w384, "Message Queue"=w382) -> ("error out"=w383:errorcluster)  [unwired: 9 in]
      n177 = call "Module Name--constant.vi"("Module ID"=w385) -> ("Module Name"=w390:string)  [unwired: 10 in]
      n178 = Format Into String(format string="An error occurred during initialization. %s is no longer running.", w390) -> (resulting string=w388:string)  [unwired: 2 in, 1 out]
      n179 = call "Error Reported.vi"("Additional Information"=w388, "Error"=w383, "Module ID"=w385) -> ()  [unwired: 8 in, 1 out]
    }
  }
  n180 = Merge Errors(w17, w16) -> (w18:errorcluster)
  n181 = call "Close Module.vi"("error in"=w18, "Wait for stop?"=w2, "Module Admin in"=w4) -> ("error out"=w14:errorcluster, "External Launch"=w1:bool, "Module Admin out"=w3:refnum<class "Delacor_lib_QMH_Cloneable Module Admin.lvclass">)  [unwired: 6 in]
  n182 = Unregister For Events(event registration refnum=w9, error in=w14) -> (error out=w13:errorcluster)
  "error out" <- w13
  n183 = local write "Module Admin"(w3) -> ()
  n184 = case "External Launch?" shown="True" w1 {
    tunnel: w13 -> [_ w392]
    frame False {
    }
    frame True {
      n185 = case shown="No Error" w392 {
        frame No Error {
          n186 = invoke class="VI" method="FP.Close"() -> ()  [unwired: 3 in, 3 out]
        }
        frame Error {
          n187 = invoke class="VI" method="FP.Open"("Activate"=TRUE ("Activate?")) -> ()  [unwired: 4 in, 5 out]
        }
      }
    }
  }
